vi "Agilent 3458 Acquire And Chart External Triggered.vi"() -> ()   [LabVIEW 2020, in "3458A Virtual Digitizer.lvlib" / "3458A Basic Driver.lvlib"]
doc: "Acquires and charts measurements taken by an external trigger. Math functions are not implemented in this VI but can be included by the user."
uses:
  3458A Basic Driver.lvlib
  Public/Data/Read Measurement(Multiple Points).vi
panel:
  in  "Manual Range (1.00)":dbl=1.0 format="%_3g"
  in  "Maximum Time (10000 ms)":u32=10000
  in  "Trigger Count (1)":dbl=1.0
  in  "Polarity (0:Negative)":u16(ring) items=["Negative", "Positive"]
  in  "Trigger Type (2:Input Complete)":u16(ring)=2 items=["Aperture Waveform", "Burst Complete", "Input Complete", "Off", "Once", "Reading Complete", "Service Request"]
  in  "Sample Count (1)":dbl=10.0 format="%#.6g"
  in  "Auto Range (1:ON)":u16(ring)=1 items=["OFF", "ON", "ONCE"]
  in  "Frequency Source (3: AC Voltage)":u16(ring)=3 items=["AC + DC Current", "AC + DC Voltage", "AC Current", "AC Voltage"]
  in  "Manual Resolution (2: 6.5 digits)":enum16{"4.5", "5.5", "6.5", "7.5", "8.5"}(ring)=enum."6.5"
  out "Waveform Chart":sgl[](graph)
  in  "Function (0: DC Voltage)":u16(ring) items=["DC Voltage", "AC Voltage", "AC + DC Voltage", "DC Current", "AC Current", "AC + DC Current", "2-Wire Resistance", "4-Wire Resistance", "Frequency", "Period", "Direct Sampling DC", "Direct Sampling AC"]
  in  "VISA resource name":refnum<visa-resource-name>
  # "(c) 2007  National Instruments.  ALL RIGHTS RESERVED."
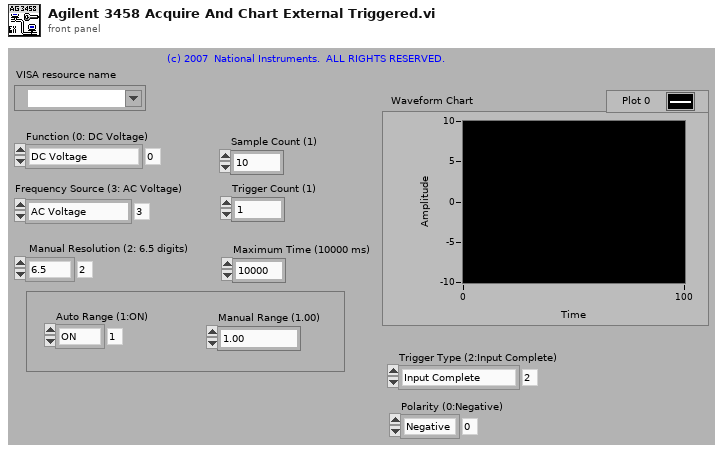
[diagram p1: front panel]
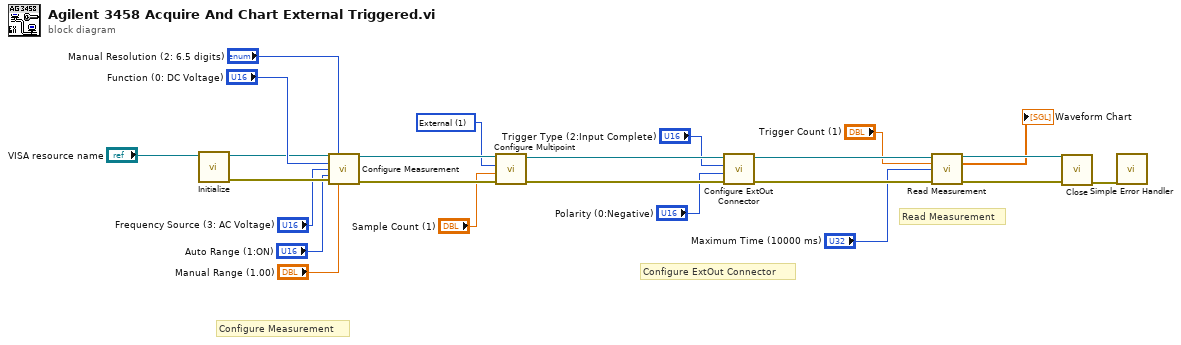
[diagram p0: block diagram]
diagram:
  w14 = u16 1 items=["Auto", "External", "Level", "Line", "Synchronous"] ("Trigger  Event(0:Auto)")
  # "Read Measurement"
  # "Configure ExtOut Connector"
  # "Configure Measurement"
  n1 = call "Initialize.vi"("VISA resource name"="VISA resource name") -> ("error out"=w12:errorcluster, "VISA resource name out"=w13:refnum<visa-resource-name>)  [unwired: 8 in, 1 out]
  n2 = call "Configure Measurement.vi"("VISA resource name"=w13, "Manual Resolution (2: 6.5 digits)"="Manual Resolution (2: 6.5 digits)", "Function (0: DC Voltage)"="Function (0: DC Voltage)", "Frequency Source (3: AC Voltage)"="Frequency Source (3: AC Voltage)", "Auto Range (1:ON)"="Auto Range (1:ON)", "error in (no error)"=w12, "Manual Range (1.00)"="Manual Range (1.00)") -> ("VISA resource name out"=w18:refnum<visa-resource-name>, "error out"=w17:errorcluster)  [unwired: 7 in]
  n3 = call "Configure Multipoint.vi"("error in (no error)"=w17, "Sample Count (1)"="Sample Count (1)", "Trigger Type (0:Auto)"=w14, "VISA resource name"=w18) -> ("error out"=w15:errorcluster, "VISA resource name out"=w16:refnum<visa-resource-name>)  [unwired: 6 in]
  n4 = call "Configure ExtOut Connector.vi"("error in (no error)"=w15, "Polarity (0:Negative)"="Polarity (0:Negative)", "Trigger Type (2:Input Complete)"="Trigger Type (2:Input Complete)", "VISA resource name"=w16) -> ("error out"=w9:errorcluster, "VISA resource name out"=w10:refnum<visa-resource-name>)  [unwired: 6 in]
  n5 = call-poly "Read Measurement.vi"("VISA resource name"=w10, "Trigger Count (1)"="Trigger Count (1)", "Maximum Time (10000 ms)"="Maximum Time (10000 ms)", "error in (no error)"=w9) -> ("VISA resource name out"=w24:refnum<visa-resource-name>, "Measurements"=→"Waveform Chart":sgl[], "error out"=w23:errorcluster)  [unwired: 9 in]
  n6 = call "Close.vi"("error in (no error)"=w23, "VISA resource name"=w24) -> ("error out"=w22:errorcluster)  [unwired: 9 in]
  n7 = call <vilib>:"Simple Error Handler.vi"("error in (no error)"=w22) -> ()  [unwired: 4 in, 5 out]
